vi "Main.vi"() -> ()   [LabVIEW 2016]
uses:
  Com/SECS Equipment/Data Def/Com_SECS Equipment _Connection Setting.ctl
  Com/SECS Equipment/Data Def/Com_SECS Equipment _Timeout Setting.ctl
panel:
  in  "Send":bool
  in  "Message":enum16{"S1F1"}(ring)
  in  "Write Tree":string(tree)
  in  "Read Tree":string(tree)
  in  "Stop":bool
  in  "Timeout Setting":T1={"T3(Reply Timeout)"=45.0, "T5(Separation Timeout)"=10.0, "T6(Control Timeout)"=5.0, "T7(Not Selected Timeout)"=10.0, "T8(Inter-Character Timeout)"=5.0}
  in  "Connection Setting":T2={"IP Address"="127.0.0.1", "Port"=5000, "Server ID"=0, "Client ID"=1}
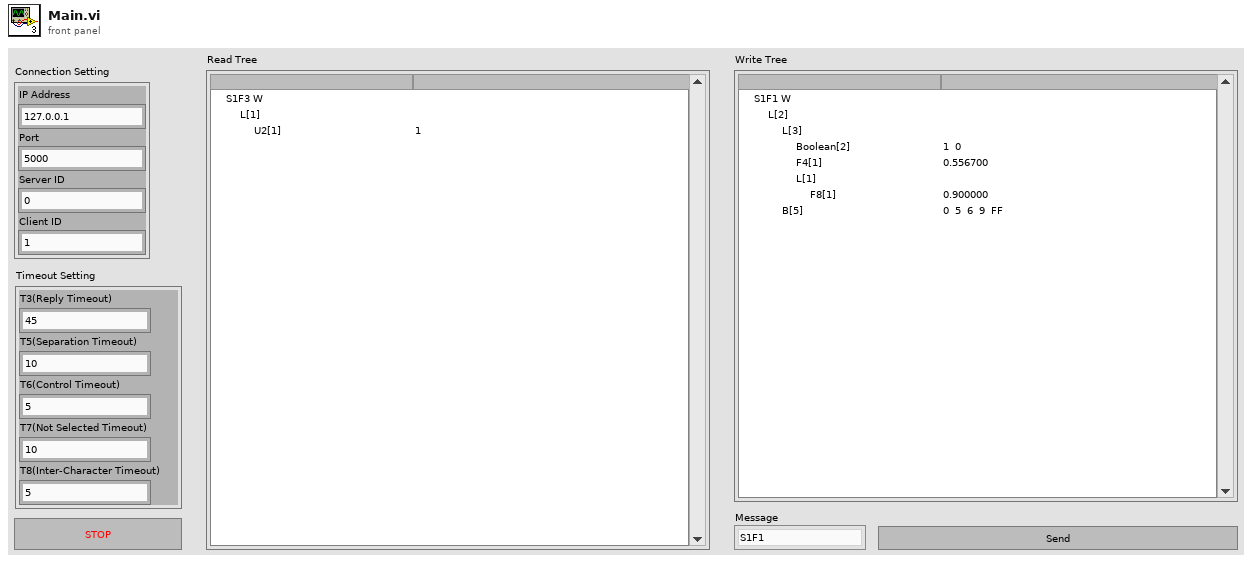
[diagram p1: front panel]
types:
  T1 = typedef "Com_SECS Equipment _Timeout Setting.ctl" = cluster{"T3(Reply Timeout)":dbl, "T5(Separation Timeout)":dbl, "T6(Control Timeout)":dbl, "T7(Not Selected Timeout)":dbl, "T8(Inter-Character Timeout)":dbl}
  T2 = typedef "Com_SECS Equipment _Connection Setting.ctl" = cluster{"IP Address":string, "Port":u16, "Server ID":u16, "Client ID":u16}
  T3 = typedef "Com_SECS Equipment _Buffer Data.ctl" = cluster{"Connection Setting":T2, "Session":cluster{"Connection ID":refnum<k5>, "Timeout Setting Notifier":refnum<notifier>}}
  T4 = typedef "Com_SECS Equipment _SECS Packet.ctl" = cluster{"Need Response?":bool, "Device ID":u16, "Stream":u8, "Function":u8, "Message Type":T5, "Protocol Type":T6, "Stream Type":T7, "System Btyes":u8[], "Message Data":u8[]}
  T5 = typedef "Com_SECS Equipment _Message Type.ctl" = enum16{"Control Message", "Data Message"}
  T6 = typedef "Com_SECS Equipment _Protocol Type.ctl" = enum16{"SECS-II Encoding", "Reserved"}
  T7 = typedef "Com_SECS Equipment _Stream Type.ctl" = enum16{"Data Message", "Select.req", "Select.rsp", "Deselect.req", "Deselect.rsp", "Linktest.req", "Linktest.rsp", "Reject.req", "Separate.req", "Reserve"}
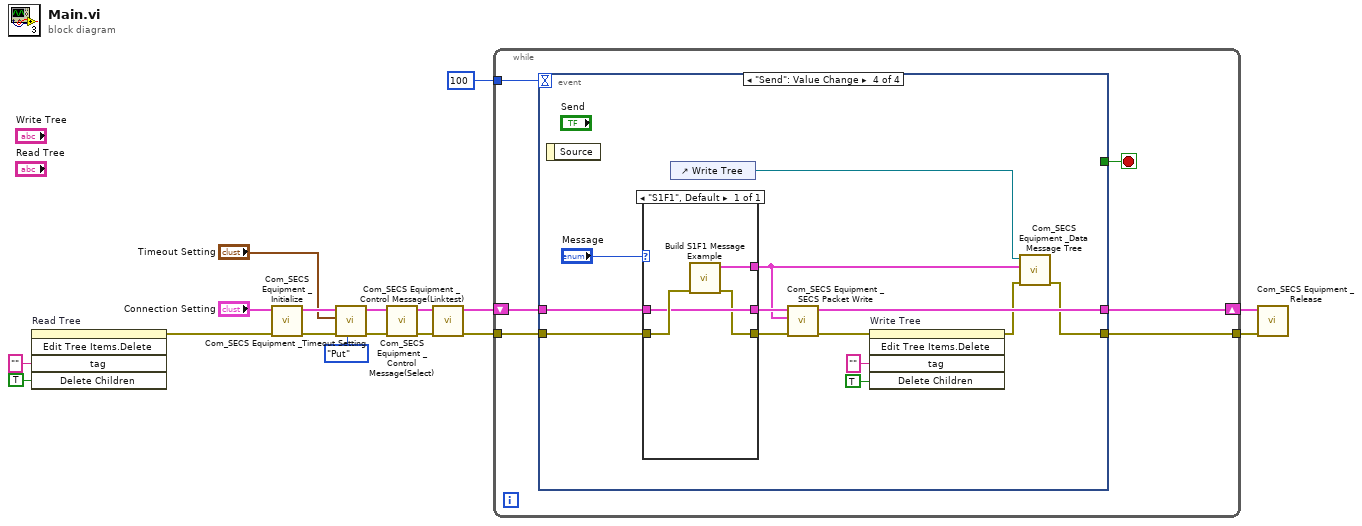
[diagram p0: block diagram]
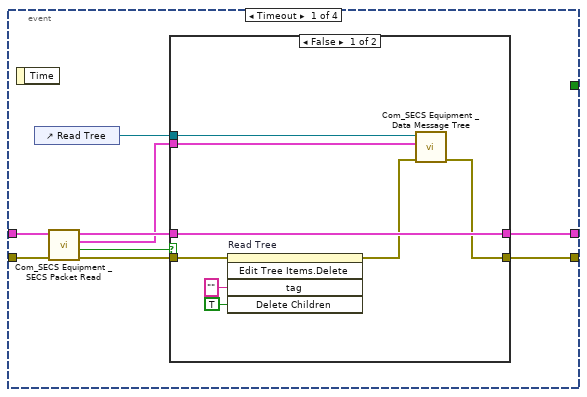
[diagram p2: hidden frame]
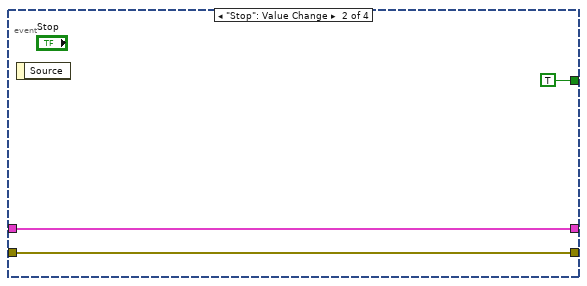
[diagram p4: hidden frame]
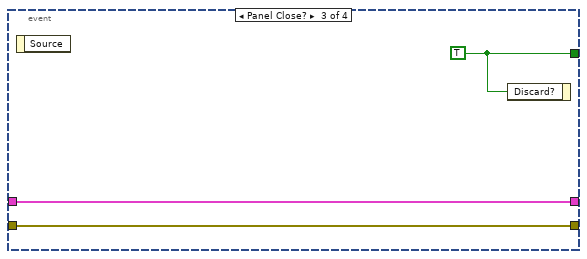
[diagram p5: hidden frame]
diagram:
  n1 = invoke on="Read Tree" class="Tree (strict)" method="Edit Tree Items.Delete"("tag"="" ("Tag"), "Delete Children"=TRUE ("Delete Children?")) -> (error out=w3:errorcluster)  [unwired: 3 in, 4 out]
  n2 = call "Com_SECS Equipment _Initialize.vi"("error in"=w3, "Connection Setting"="Connection Setting") -> ("error out"=w1:errorcluster, "Buffer Data"=w16:T3)  [unwired: 8 in]
  n3 = call "Com_SECS Equipment _Timeout Setting.vi"("Method"=enum16{"Get", "Put"}."Put", "error in"=w1, "Timeout Setting In"="Timeout Setting", "Buffer Data In"=w16) -> ("error out"=w12:errorcluster, "Buffer Data Out"=w13:T3)  [unwired: 5 in, 1 out]
  n4 = call "Com_SECS Equipment _Control Message(Select).vi"("error in"=w12, "Buffer Data In"=w13) -> ("error out"=w10:errorcluster, "Buffer Data Out"=w11:T3)  [unwired: 8 in]
  n5 = call "Com_SECS Equipment _Control Message(Linktest).vi"("error in"=w10, "Buffer Data In"=w11) -> ("error out"=w9:errorcluster, "Buffer Data Out"=w8:T3)  [unwired: 8 in]
  n6 = while {
    tunnel: w9 -> [w23]
    shift-right: [w21] -> w6
    shift-left: w8 -> [w22]
    tunnel: [w20] -> w7
    tunnel: 100 -> [w19]
    stop <- w18 stop-if-true
    n7 = event shown="[3] \"Send\": Value Change" {
      selector: _ -> [_ _ _ _]
      dyn-events: _ -> [_ _ _ _]
      timeout: w19 -> [_ _ _ _]
      tunnel: w23 -> [w32 w43 w46 w59]
      tunnel: w22 -> [w31 w44 w47 w58]
      tunnel: [w27 w44 w47 w55] -> w21
      tunnel: [w25 w43 w46 w53] -> w20
      tunnel: [_ TRUE w45 _] -> w18
      event Timeout {
        n8 = event-data() -> ()  [unwired: 1 in, 1 out]
        n9 = control-ref of="Read Tree"() -> (w24:refnum<vi>)
        n10 = call "Com_SECS Equipment _SECS Packet Read.vi"("error in"=w32, "Buffer Data In"=w31) -> ("error out"=w30:errorcluster, "Timeout?"=w29:bool, "SECS Packet"=w26:T4, "Buffer Data Out"=w28:T3)  [unwired: 6 in]
        n11 = case shown="False" w29 {
          tunnel: w30 -> [w39 _]
          tunnel: w28 -> [w40 w41]
          tunnel: [w40 w41] -> w27
          tunnel: w26 -> [w35 _]
          tunnel: [w33 _] -> w25
          tunnel: w24 -> [w34 _]
          frame False {
            n12 = invoke on="Read Tree" class="Tree (strict)" method="Edit Tree Items.Delete"(error in=w39, "tag"="" ("Tag"), "Delete Children"=TRUE ("Delete Children?")) -> (error out=w36:errorcluster)  [unwired: 2 in, 4 out]
            n13 = call "Com_SECS Equipment _Data Message Tree.vi"("error in"=w36, "SECS Packet"=w35, "Tree Refnum"=w34) -> ("error out"=w33:errorcluster)  [unwired: 8 in]
          }
          frame True {
          }
        }
      }
      event "Stop": Value Change {
        n14 = event-data() -> ()  [unwired: 1 in, 1 out]
      }
      event Panel Close? {
        w45 = TRUE
        n15 = event-data() -> ()  [unwired: 1 in, 1 out]
        n16 = event-data("Discard?"=w45) -> ()  [unwired: 1 in, 1 out]
      }
      event "Send": Value Change {
        n17 = event-data() -> ()  [unwired: 1 in, 1 out]
        n18 = case shown="\"S1F1\", Default" "Message" {
          tunnel: w59 -> [w64]
          tunnel: w58 -> [w63]
          tunnel: [w63] -> w56
          tunnel: [w62] -> w57
          tunnel: [w61] -> w54
          frame "S1F1", Default {
            n19 = call "Build S1F1 Message Example.vi"("error in"=w64) -> ("error out"=w62:errorcluster, "SECS Packet"=w61:T4)  [unwired: 9 in]
          }
        }
        n20 = control-ref of="Write Tree"() -> (w52:refnum<vi>)
        n21 = call "Com_SECS Equipment _SECS Packet Write.vi"("error in"=w57, "SECS Packet"=w54, "Buffer Data In"=w56) -> ("error out"=w51:errorcluster, "Buffer Data Out"=w55:T3)  [unwired: 7 in]
        n22 = invoke on="Write Tree" class="Tree (strict)" method="Edit Tree Items.Delete"(error in=w51, "tag"="" ("Tag"), "Delete Children"=TRUE ("Delete Children?")) -> (error out=w50:errorcluster)  [unwired: 2 in, 4 out]
        n23 = call "Com_SECS Equipment _Data Message Tree.vi"("error in"=w50, "SECS Packet"=w54, "Tree Refnum"=w52) -> ("error out"=w53:errorcluster)  [unwired: 8 in]
      }
    }
  }
  n24 = call "Com_SECS Equipment _Release.vi"("error in"=w7, "Buffer Data"=w6) -> ()  [unwired: 9 in, 1 out]
